vi "delete profile.vi"   [LabVIEW 2010]
uses:
  SubVIs/Watflow F4/Watflow F4.lvlib
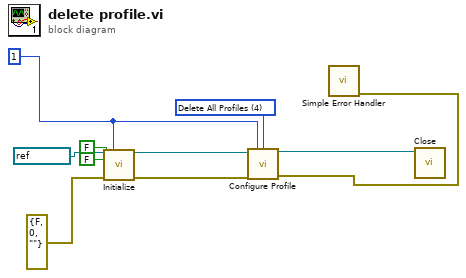
[diagram p0: block diagram]
diagram:
  w7 = u8 1 ("Unit Address (1)")
  w10 = u16 4 items=["Create Profile", "Delete Current Profile", "Delete Step", "Start Profile", "Delete All Profiles", "Rename Profile"] ("Action (0: Create Profile)")
  n1 = call "Initialize.vi"("VISA resource name"=refnum<visa-resource-name> "COM3", "Unit Address (1)"=w7, "ID Query (T: Check)"=FALSE, "Reset (T: Reset)"=FALSE, "error in (no error)"=errorcluster {"status"=FALSE, "code"=0, "source"=""}) -> ("VISA resource name out"=w9:refnum<visa-resource-name>, "error out"=w8:errorcluster)  [unwired: 9 in]
  n2 = call "Configure Profile.vi"("VISA resource name"=w9, "Unit Address (1)"=w7, "Action (0: Create Profile)"=w10, "error in (no error)"=w8) -> ("VISA resource name out"=w4:refnum<visa-resource-name>, "error out"=w3:errorcluster)  [unwired: 10 in]
  n3 = call <vilib>:"Simple Error Handler.vi"("error in (no error)"=w3) -> ()  [unwired: 4 in, 5 out]
  n4 = call "Close.vi"("VISA resource name"=w4) -> ()  [unwired: 14 in, 1 out]
